vi "Handle Command.vi"(8 "error in (no error)":errorcluster, 10 "CMD in":refnum<class "Update Laser rate and DC.lvclass">, 11 "Object In":refnum<class>) -> (0 "error out":errorcluster, 1 "Command Successful?":bool, 2 "CMD out":refnum<class "Update Laser rate and DC.lvclass">, 3 "Object Out":refnum<class>)   [LabVIEW 2014, in "eCRDS Library.lvlib" / "Update Laser rate and DC.lvclass"]
doc: "This VI will contain the code used to actually execute the request. If the request is successful, this will be indicated by the boolean output <b>Command Successful?</b>. The boolean output can then be used by the <b>Command Reply</b> which sends a reply if the reply queue is valid."
uses:
  Update Laser rate and DC.lvclass
  Main/eCRDS.lvclass
  Main/eCRDS.lvclass/eCRDS.ctl
  reusable/Instrument/Instrument.lvclass/Instrument.ctl
  Update Laser rate and DC.lvclass/Update Laser rate and DC.ctl
  Main/Accessors/Read DAQ.vi
  Main/Accessors/Read Tasks.vi
  reusable/Instrument/Read Log Session.vi
  Main/Accessors/Write DAQ.vi
  <userlib>/_Session Fwk/Session - Root.lvclass
  reusable/Session APIs/Session Log/System Log.lvclass
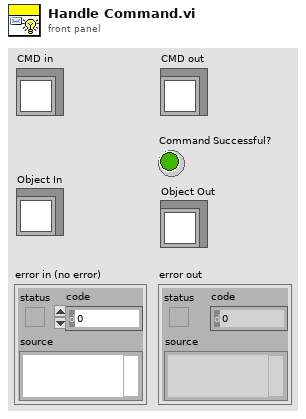
[diagram p1: front panel]
types:
  T1 = cluster{"Rate (MHz)":dbl, "Laser Rep (Hz)":dbl, "Laser DC (%)":dbl}
  T2 = cluster{"CLk":refnum<k21>, "AI":refnum<k21>, "DO":refnum<k21>}
  T3 = typedef "Session - Root.lvclass/Session Handle.ctl" = refnum<data-value>
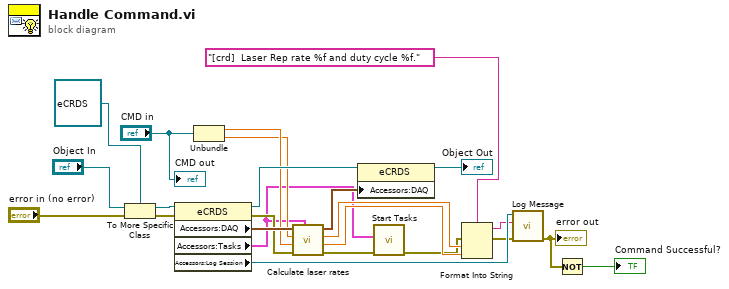
[diagram p0: block diagram]
diagram:
  n1 = To More Specific Class(target class=refnum<class "eCRDS.lvclass"> refnum ("eCRDS"), reference="Object In", error in="error in (no error)") -> (specific class reference=w24:refnum<class "eCRDS.lvclass">, error out=w23:errorcluster)
  n2 = property class="eCRDS"(reference=w24, error in=w23) -> (reference out=w22:refnum<class "eCRDS.lvclass">, error out=w5:errorcluster, "Accessors:DAQ"=w11:T1, "Accessors:Tasks"=w4:T2, "Accessors:Log Session"=w21:T3)
  n3 = Unbundle("CMD in") -> (w10:dbl, w9:dbl)
  n4 = call "Calculate laser rates.vi"("Tasks"=w4, "error in (no error)"=w5, "Laser DC (%)"=w10, "Laser Rep (Hz)"=w9, "DAQ"=w11) -> ("error out"=w1:errorcluster, "Laser DC"=w6:dbl, "Laser Rep (Hz)"=w7:dbl, "DAQ"=w8:T1)  [unwired: 3 in]
  n5 = property class="eCRDS"(reference=w22, "Accessors:DAQ"=w8) -> (reference out=→"Object Out":refnum<class "eCRDS.lvclass">)  [unwired: 1 in, 1 out]
  n6 = call "Start Tasks.vi"("error in"=w1, "Red Tasks"=w4) -> ("error out"=w3:errorcluster)  [unwired: 9 in]
  n7 = Format Into String(format string="[crd]  Laser Rep rate %f and duty cycle %f.", error in=w3, w7, w6) -> (resulting string=w19:string, error out=w18:errorcluster)  [unwired: 1 in]
  n8 = call "Log Message.vi"("error in"=w18, "MSG In"=w19, "session in"=w21) -> ("error out"=w2:errorcluster)  [unwired: 7 in, 1 out]
  "error out" <- w2
  n9 = Not(x=w2) -> (.not. x?=→"Command Successful?":bool)
  "CMD out" <- "CMD in"
